vi "WSVCAP SHL Host TL Status Manager.vi"(0 "System In":T2={"Settings"={"FPGA Resource Name"="", "I2C Slave Address"=20, "I2C Clock Rate (Hz)"=50000.0, "SPI Clock Rate (Hz)"=50000.0, "RFFE Slave Address"=20, "RFFE Clock Rate (Hz)"=50000.0, "Simulate FPGA"=TRUE}, "FPGA Resource"="", "Online"=FALSE, "I2C Wait Ticks"=0, "SPI Wait Ticks"=0, "RFFE Wait Ticks"=0} {"Settings"."RFFE Clock Rate (Hz)" format="%.0f Hz"; "Settings"."RFFE Slave Address" format="0x%02x"; "Settings"."I2C Clock Rate (Hz)" format="%.0f Hz"; "Settings"."SPI Clock Rate (Hz)" format="%.0f Hz"; "Settings"."I2C Slave Address" format="0x%02x"}, 11 "error in":errorcluster, 13 "Operation (Read)":T1) -> (4 "System Out":T2={"Settings"={"FPGA Resource Name"="", "I2C Slave Address"=20, "I2C Clock Rate (Hz)"=50000.0, "SPI Clock Rate (Hz)"=50000.0, "RFFE Slave Address"=20, "RFFE Clock Rate (Hz)"=50000.0, "Simulate FPGA"=TRUE}, "FPGA Resource"="", "Online"=FALSE, "I2C Wait Ticks"=0, "SPI Wait Ticks"=0, "RFFE Wait Ticks"=0} {"Settings"."RFFE Clock Rate (Hz)" format="%.0f Hz"; "Settings"."RFFE Slave Address" format="0x%02x"; "Settings"."I2C Clock Rate (Hz)" format="%.0f Hz"; "Settings"."SPI Clock Rate (Hz)" format="%.0f Hz"; "Settings"."I2C Slave Address" format="0x%02x"}, 15 "error out":errorcluster)   [LabVIEW 2012]
uses:
  Type Defs/WSVCAP SHL Core System Cluster.ctl
  Type Defs/WSVCAP SHL I2C Settings Cluster.ctl
  user.lib/Utilities/Type Defs/MISC IO Choice Enum.ctl
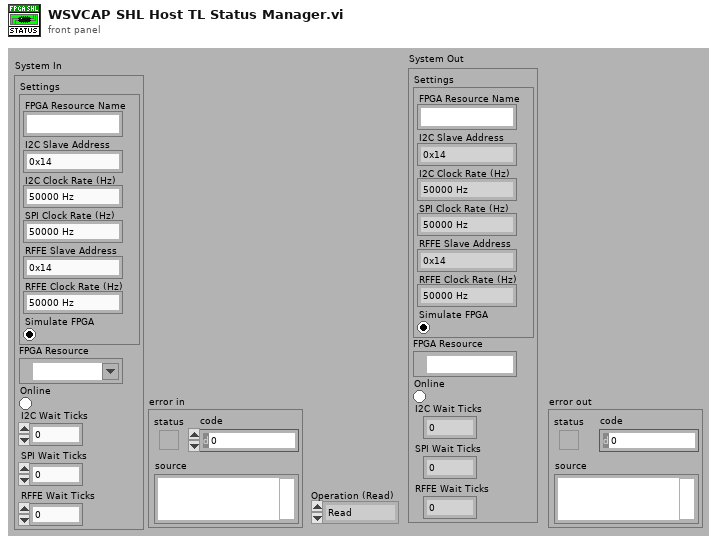
[diagram p1: front panel]
types:
  T1 = typedef "MISC IO Choice Enum.ctl" = enum16{"Read", "Write"}
  T2 = typedef "WSVCAP SHL Core System Cluster.ctl" = cluster{"Settings":T3, "FPGA Resource":tag, "Online":bool, "I2C Wait Ticks":u32, "SPI Wait Ticks":u32, "RFFE Wait Ticks":u32}
  T3 = typedef "WSVCAP SHL I2C Settings Cluster.ctl" = cluster{"FPGA Resource Name":string, "I2C Slave Address":u8, "I2C Clock Rate (Hz)":dbl, "SPI Clock Rate (Hz)":dbl, "RFFE Slave Address":u8, "RFFE Clock Rate (Hz)":dbl, "Simulate FPGA":bool}
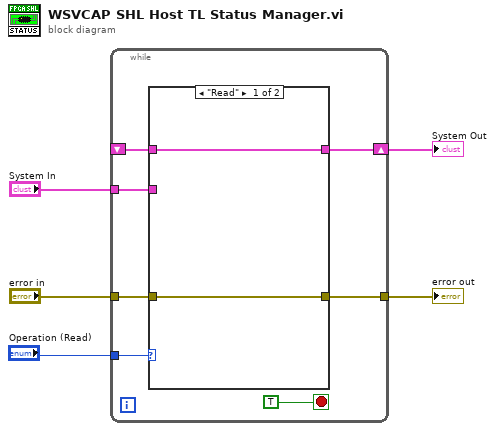
[diagram p0: block diagram]
diagram:
  n1 = while {
    tunnel: "Operation (Read)" -> [w11]
    tunnel: "error in" -> [w10]
    tunnel: [w9] -> w4
    shift-right: [w8] -> w3
    shift-left: _ -> [w7]
    tunnel: "System In" -> [w6]
    stop <- TRUE ("stop") stop-if-true
    n2 = case shown="\"Read\"" w11 {
      tunnel: w10 -> [w14 w16]
      tunnel: [w14 w16] -> w9
      tunnel: [w13 w15] -> w8
      tunnel: w7 -> [w13 _]
      tunnel: w6 -> [_ w15]
      frame "Read" {
      }
      frame "Write" {
      }
    }
  }
  "error out" <- w4
  "System Out" <- w3
